vi "Read Outgoing Work Dispatcher.vi"(8 "error in (no error)":errorcluster, 11 "Worker In":refnum<class "Worker.lvclass">) -> (0 "error out":errorcluster, 2 "Job Handler":refnum<class "Job Handler.lvclass">, 3 "Worker Out":refnum<class "Worker.lvclass">)   [LabVIEW 2020, in "Worker.lvclass"]
uses:
  Worker.lvclass
  Process Job/Job Handler.lvclass
  Worker.lvclass/Worker.ctl
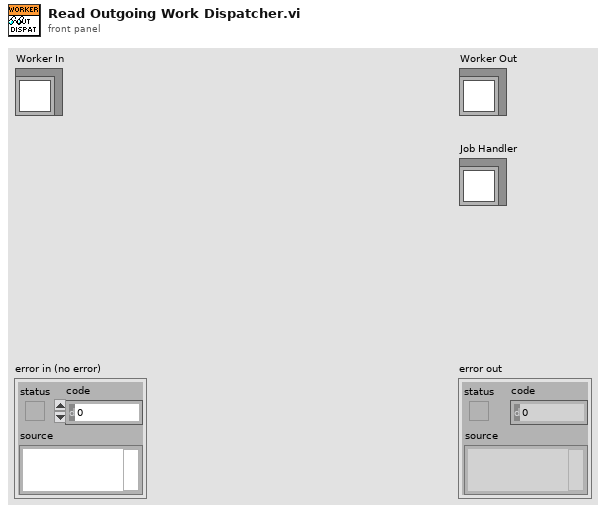
[diagram p1: front panel]
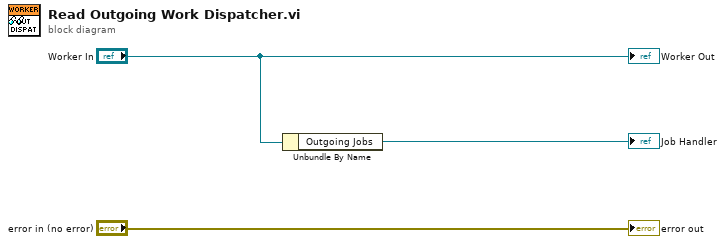
[diagram p0: block diagram]
diagram:
  n1 = Unbundle By Name("Worker In") -> ("Outgoing Jobs"=→"Job Handler":refnum<class "Job Handler.lvclass">)
  "error out" <- "error in (no error)"
  "Worker Out" <- "Worker In"
